vi "VI Snippet Dialog.vi"(8 "error in (no error)":errorcluster, 11 "VI Snippets Dir":path) -> (0 "error out":errorcluster, 1 "Cancelled?":bool, 2 "New VI?":bool, 3 "VI Snippets Path":path)   [LabVIEW 2019, in "VI Snippet.lvlib"]
doc: "Opens a dialog window to preview and select a VI Snippet (*.png) from the list of images located in the <b>VI Snippet Dir</b>. Large images are scaled to fit.\n\nCreated By: Ryan Pacini"
uses:
  VI Snippet.lvlib
panel:
  in  "Filename":u16(ring) items=["basic.png", "broken_wires_only.png", "crc32_lookup_table.png", "decorations_only.png", "example.png", "fg.png", "large.png", "missing_terminal.png", "sub_vi_missing.png", "VI Tree.png", "vi_lib_dependency.png"]
  in  "Copy to Clipboard":bool
  in  "Cancel":bool
  in  "Copy to New VI":bool
  out "Preview":picture
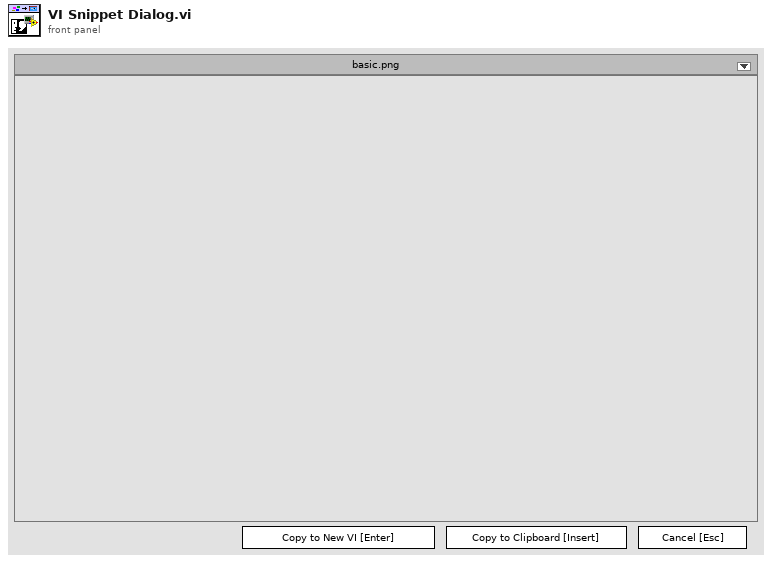
[diagram p1: front panel]
types:
  T1 = typedef "imagedata.ctl" = cluster{"image type":i32, "image depth":i32, "image":u8[], "mask":u8[], "colors":u32[], "Rectangle":cluster{"left":i16, "top":i16, "right":i16, "bottom":i16}}
  T2 = typedef "LVBoundsTypeDef.ctl" = cluster{"Width":u32, "Height":u32}
  T3 = cluster{"left":i16, "top":i16, "right":i16, "bottom":i16}
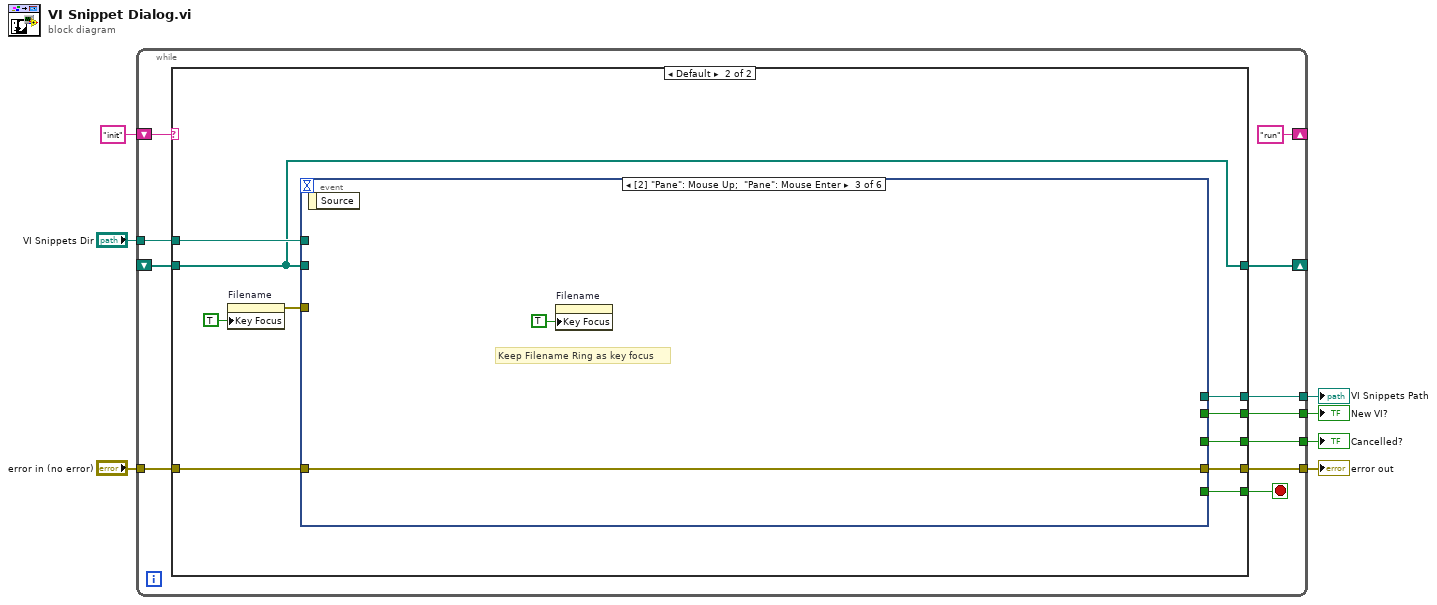
[diagram p0: block diagram]
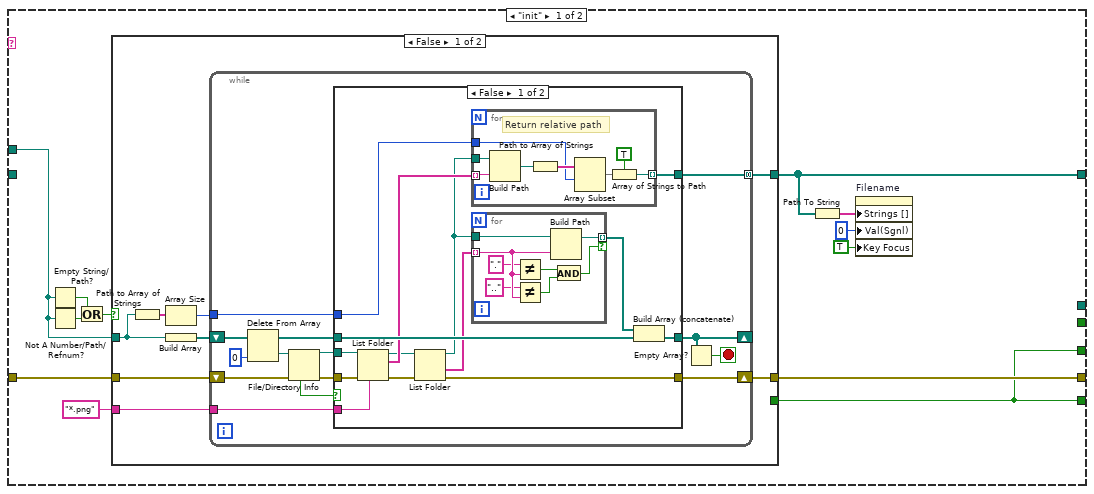
[diagram p2: hidden frame]
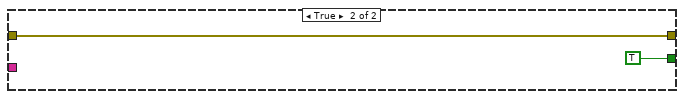
[diagram p4: hidden frame]
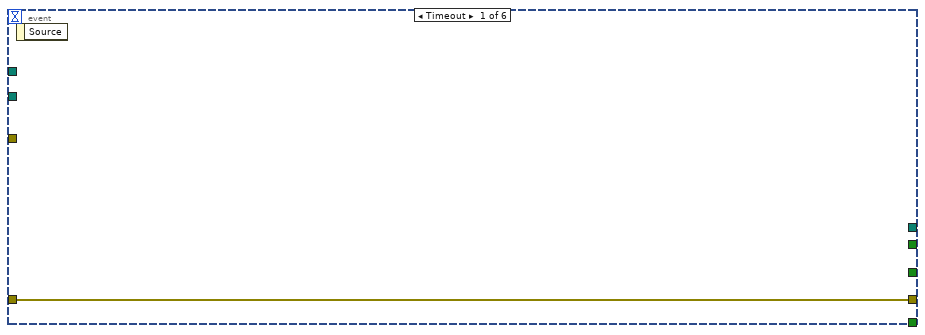
[diagram p5: hidden frame]
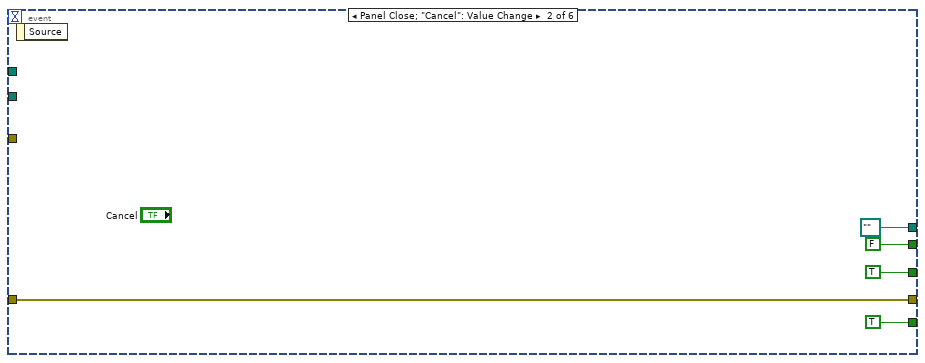
[diagram p6: hidden frame]
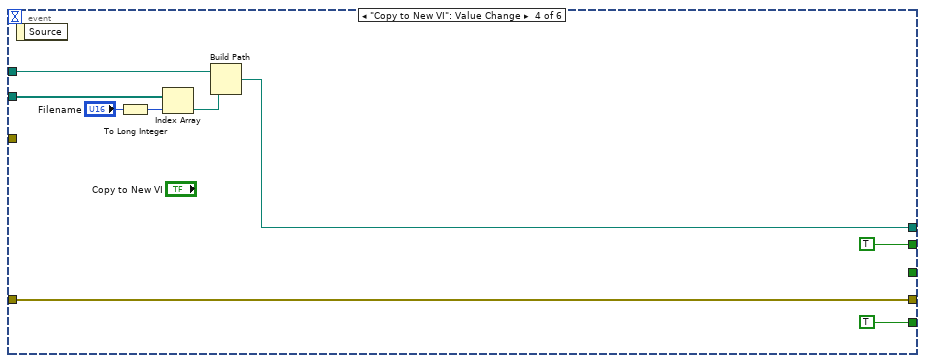
[diagram p7: hidden frame]
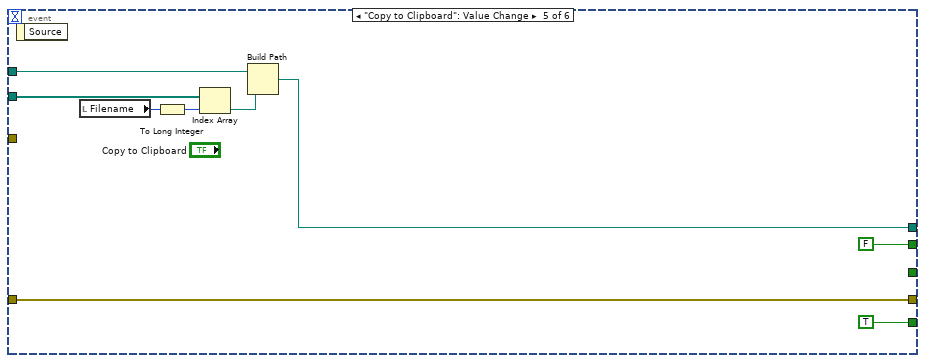
[diagram p8: hidden frame]
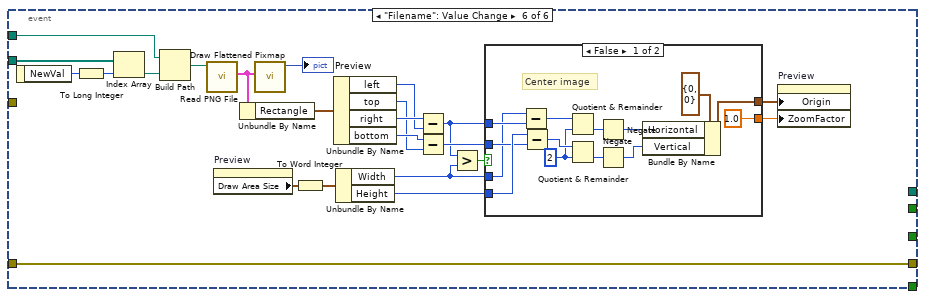
[diagram p9: hidden frame]
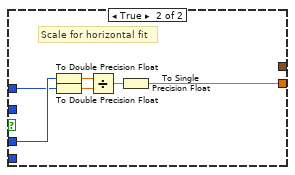
[diagram p10: hidden frame]
diagram:
  n1 = while {
    tunnel: [w18] -> w7
    tunnel: "error in (no error)" -> [w17]
    tunnel: [w15] -> w5
    tunnel: [w14] -> w6
    shift-right: ["run"] -> _
    shift-left: "init" -> [w13]
    tunnel: "VI Snippets Dir" -> [w11]
    shift-right: [w10] -> _
    shift-left: _ -> [w9]
    tunnel: [w8] -> w2
    stop <- w16 stop-if-true
    n2 = case shown="Default" w13 {
      tunnel: [w21 w96] -> w18
      tunnel: w17 -> [w23 w95]
      tunnel: [w19 w94] -> w16
      tunnel: [_ w93] -> w15
      tunnel: [_ w92] -> w14
      tunnel: w11 -> [w22 w89]
      tunnel: [w20 w88] -> w10
      tunnel: w9 -> [_ w88]
      tunnel: [w19 w87] -> w8
      frame "init" {
        n3 = Empty String/Path?(string/path=w22) -> (empty?=w28:bool)
        n4 = Not A Number/Path/Refnum?(number/path/refnum=w22) -> (NaN/Path/Refnum?=w27:bool)
        n5 = Or(x=w28, y=w27) -> (x .or. y?=w29:bool)
        n6 = case shown="False" w29 {
          tunnel: w23 -> [w38 w86]
          tunnel: "*.png" ("pattern") -> [w37 _]
          tunnel: [w36 w86] -> w21
          tunnel: [w34 _] -> w20
          tunnel: w22 -> [w31 _]
          tunnel: [_ TRUE] -> w19
          frame False {
            n7 = Path to Array of Strings(0:w31) -> (2:w33:string[])  [unwired: 1 out]
            n8 = Array Size(array=w33) -> (size(s)=w32:i32)
            n9 = Build Array(w31) -> (w35:path[])
            n10 = while {
              shift-left: w35 -> [w52]
              shift-right: [w50] -> _
              shift-right: [w47] -> w36
              shift-left: w38 -> [w45]
              tunnel: w37 -> [w51]
              tunnel: [w42] -> w34 mode=concatenating
              tunnel: w32 -> [w39]
              stop <- w49 stop-if-true
              n11 = Delete From Array(array=w52, index=0) -> (deleted portion=w41:path, array with subset deleted=w46:path[])  [unwired: 1 in]
              n12 = File/Directory Info(path=w41, error in=w45) -> (path out=w40:path, error out=w44:errorcluster, shortcut=w43:bool)  [unwired: 4 out]
              n13 = case shown="False" w43 {
                tunnel: w51 -> [w66 _]
                tunnel: [w65 w84] -> w50
                tunnel: [w64 w83] -> w47
                tunnel: w46 -> [w63 w84]
                tunnel: w44 -> [w61 w83]
                tunnel: [w58 _] -> w42
                tunnel: w40 -> [w54 _]
                tunnel: w39 -> [w53 _]
                frame False {
                  n14 = List Folder(path=w54, pattern=w66, error in=w61) -> (path out=w57:path, filenames=w60:string[], error out=w56:errorcluster)  [unwired: 2 out]
                  n15 = List Folder(path=w57, error in=w56) -> (path out=w55:path, folder names=w62:string[], error out=w64:errorcluster)  [unwired: 3 out]
                  n16 = for {
                    tunnel: w60 -> [w81] mode=indexing
                    tunnel: w55 -> [w82]
                    tunnel: [w76] -> w58 mode=indexing
                    tunnel: w53 -> [w78]
                    # "Return relative path"
                    n17 = Build Path(base path=w82, name or relative path=w81) -> (appended path=w80:path)
                    n18 = Path to Array of Strings(0:w80) -> (2:w79:string[])  [unwired: 1 out]
                    n19 = Array Subset(array=w79, index=w78) -> (w77:string[])  [unwired: 1 in]
                    n20 = Array of Strings to Path(0:w77, 1:TRUE ("relative")) -> (2:w76:path)
                  }
                  n21 = for {
                    tunnel: w55 -> [w74]
                    tunnel: [w73] -> w59 mode=indexing if=w72
                    tunnel: w62 -> [w71] mode=indexing
                    n22 = Not Equal?(x="." ("y"), y=w71) -> (x != y?=w69:bool)
                    n23 = Not Equal?(x=".." ("y"), y=w71) -> (x != y?=w70:bool)
                    n24 = Build Path(base path=w74, name or relative path=w71) -> (appended path=w73:path)
                    n25 = And(x=w69, y=w70) -> (x .and. y?=w72:bool)
                  }
                  n26 = Build Array (concatenate)(w59, w63) -> (w65:path[])
                }
                frame True {
                }
              }
              n27 = Empty Array?(array=w50) -> (empty?=w49:bool)
            }
          }
          frame True {
          }
        }
        n28 = Path To String(path=w20) -> (string=w30:string[])
        n29 = property on="Filename" class="Ring (strict)"("Strings []"=w30, "Val(Sgnl)"=u16 0 ("Value (Signaling)"), "Key Focus"=TRUE) -> ()  [unwired: 2 in, 2 out]
      }
      frame Default {
        n30 = property on="Filename" class="Ring (strict)"("Key Focus"=TRUE) -> (error out=w90:errorcluster)  [unwired: 2 in, 1 out]
        n31 = event shown="[2] \"Pane\": Mouse Up;  \"Pane\": Mouse Enter" {
          selector: _ -> [_ _ _ _ _ _]
          dyn-events: _ -> [_ _ _ _ _ _]
          timeout: _ -> [_ _ _ _ _ _]
          tunnel: [w97 w102 w104 w113 w122 w145] -> w96
          tunnel: w95 -> [w97 w102 w104 w113 w122 w145]
          tunnel: w88 -> [_ _ _ w111 w120 w144]
          tunnel: w89 -> [_ _ _ w112 w121 w141]
          tunnel: [_ TRUE _ TRUE TRUE _] -> w94
          tunnel: [_ FALSE _ TRUE FALSE _] -> w93
          tunnel: [_ path "" ("VI Snippets Path") _ w107 w117 _] -> w92
          tunnel: w90 -> [_ _ _ _ _ _]
          tunnel: [_ TRUE _ _ _ _] -> w87
          event Timeout {
            n32 = event-data() -> ()  [unwired: 1 in, 1 out]
          }
          event Panel Close; "Cancel": Value Change {
            n33 = event-data() -> ()  [unwired: 1 in, 1 out]
          }
          event Mouse Up; Mouse Enter {
            # "Keep Filename Ring as key focus"
            n34 = event-data() -> ()  [unwired: 1 in, 1 out]
            n35 = property on="Filename" class="Ring (strict)"("Key Focus"=TRUE) -> ()  [unwired: 2 in, 2 out]
          }
          event "Copy to New VI": Value Change {
            n36 = event-data() -> ()  [unwired: 1 in, 1 out]
            n37 = To Long Integer(number="Filename") -> (32bit integer=w108:i32)
            n38 = Index Array(array=w111, index=w108) -> (element=w109:path)
            n39 = Build Path(base path=w112, name or relative path=w109) -> (appended path=w107:path)
          }
          event "Copy to Clipboard": Value Change {
            n40 = event-data() -> ()  [unwired: 1 in, 1 out]
            n41 = local read "Filename"() -> (w115:u16)
            n42 = To Long Integer(number=w115) -> (32bit integer=w118:i32)
            n43 = Index Array(array=w120, index=w118) -> (element=w119:path)
            n44 = Build Path(base path=w121, name or relative path=w119) -> (appended path=w117:path)
          }
          event "Filename": Value Change {
            n45 = event-data() -> ("NewVal"=w143:u16)  [unwired: 1 in]
            n46 = To Long Integer(number=w143) -> (32bit integer=w142:i32)
            n47 = Index Array(array=w144, index=w142) -> (element=w140:path)
            n48 = Build Path(base path=w141, name or relative path=w140) -> (appended path=w139:path)
            n49 = call <vilib>:"Read PNG File.vi"("path to PNG file"=w139) -> ("image data"=w136:T1)  [unwired: 8 in, 2 out]
            n50 = property on="Preview" class="Pict"() -> ("Draw Area Size"=w137:T2)  [unwired: 2 in, 2 out]
            n51 = Unbundle By Name(w136) -> ("Rectangle"=w135:T3)
            n52 = call <vilib>:"Draw Flattened Pixmap.vi"("image data"=w136) -> ("new picture"=→"Preview":picture)  [unwired: 8 in]
            n53 = To Word Integer(number=w137) -> (16bit integer=w130:cluster{"Width":i16, "Height":i16})
            n54 = Unbundle By Name(w135) -> ("left"=w131:i16, "top"=w132:i16, "right"=w134:i16, "bottom"=w133:i16)
            n55 = Unbundle By Name(w130) -> ("Width"=w125:i16, "Height"=w129:i16)
            n56 = Subtract(x=w134, y=w131) -> (x-y=w126:i16)
            n57 = Subtract(x=w133, y=w132) -> (x-y=w128:i16)
            n58 = Greater?(x=w126, y=w125) -> (0:w124:bool)
            n59 = case shown="False" w124 {
              tunnel: w129 -> [w159 _]
              tunnel: w128 -> [w158 _]
              tunnel: [w153 _] -> w127
              tunnel: w126 -> [w157 w164]
              tunnel: w125 -> [w156 w165]
              tunnel: [sgl 1.0 ("Zoom Factor") w162] -> w123
              frame False {
                w146 = i16 2 ("y")
                # "Center image"
                n60 = Subtract(x=w156, y=w157) -> (x-y=w152:i16)
                n61 = Subtract(x=w159, y=w158) -> (x-y=w150:i16)
                n62 = Quotient & Remainder(x=w152, y=w146) -> (floor(x/y)=w151:i16)  [unwired: 1 out]
                n63 = Quotient & Remainder(x=w150, y=w146) -> (floor(x/y)=w149:i16)  [unwired: 1 out]
                n64 = Negate(x=w151) -> (-x=w148:i16)
                n65 = Negate(x=w149) -> (-x=w147:i16)
                n66 = Bundle By Name(cluster=cluster{"Horizontal":i16, "Vertical":i16} {"Horizontal"=0, "Vertical"=0} ("Origin"), "Horizontal"=w148, "Vertical"=w147) -> (w153:cluster{"Horizontal":i16, "Vertical":i16})
              }
              frame True {
                # "Scale for horizontal fit"
                n67 = To Double Precision Float(number=w165) -> (double precision float=w161:dbl)
                n68 = To Double Precision Float(number=w164) -> (double precision float=w160:dbl)
                n69 = Divide(x=w161, y=w160) -> (x/y=w163:dbl)
                n70 = To Single Precision Float(number=w163) -> (single precision float=w162:sgl)
              }
            }
            n71 = property on="Preview" class="Pict"("Origin"=w127, "ZoomFactor"=w123) -> ()  [unwired: 2 in, 2 out]
          }
        }
      }
    }
  }
  "error out" <- w7
  "VI Snippets Path" <- w6
  "New VI?" <- w5
  "Cancelled?" <- w2
